vi "Main.vi"(11 "Module Admin":refnum<class "Delacor_lib_QMH_Cloneable Module Admin.lvclass">) -> ()   [LabVIEW 2021, in "MQTT Bridge.lvlib"]
doc: "This template is based off of the Queued Message Handler design pattern and the Queued Message Handler project template that ships with LabVIEW.\n\nThe main difference is that the queue is private to this module and communication between modules is performed via Broadcast and Request events.\n\nRequest events are wrapped in public API methods and are handled in the Event Handling Loop (EHL) of this VI. Any module can register for Broadcast events sent by this module. The EHL generates messages based on user interface actions.\n\nThe Message Handling Loop (MHL) processes messages generated by the EHL, or by other messages. The messages are string values, so new messages can be added easily to the Message Cases case structure in the MHL. Each message cluster can also provide an optional value for Message Data, which is a variant that can be converted to whatever message-specific data is required.\n_____\nBased on DQMH Dev Tools: Project Template 7.1.1.1528."
uses:
  MQTT Bridge.lvlib
  <vilib>/Delacor/Delacor QMH/Libraries/Cloneable Module Admin_class/Delacor_lib_QMH_Cloneable Module Admin.lvclass
  C:/Program Files (x86)/National Instruments/LabVIEW 2021/vi.lib/Delacor/Delacor QMH/Libraries/Module Admin_class/Delacor_lib_QMH_Module Admin.lvclass
  <vilib>/LabVIEW Open Source Project/MQTT Client/Client class/Client.lvclass/Client.ctl
  <vilib>/LabVIEW Open Source Project/MQTT Connection/MQTT_Base/Base Class/MQTT_Base.lvclass/MQTT_Base.ctl
  Module Data--cluster.ctl
  <vilib>/LabVIEW Open Source Project/MQTT Client/Client class/Client.lvclass
  C:/Program Files (x86)/National Instruments/LabVIEW 2021/vi.lib/LabVIEW Open Source Project/MQTT Connection/MQTT_Base/Base Class/MQTT_Base.lvclass
  <vilib>/Delacor/Delacor QMH/Libraries/Cloneable Module Admin_class/Delacor_lib_QMH_Cloneable Module Admin.lvclass/Delacor_lib_QMH_Cloneable Module Admin.ctl
  <vilib>/Delacor/Delacor QMH/Libraries/Message Queue_class/Delacor_lib_QMH_Message Queue.lvclass/Delacor_lib_QMH_Message Queue.ctl
  Stop Argument--cluster.ctl
  <vilib>/Delacor/Delacor QMH/Libraries/Module Admin_class/Delacor_lib_QMH_Module Admin.lvclass/Delacor_lib_QMH_Module Admin.ctl
  Connect Argument--cluster.ctl
  Subscribe Argument--cluster.ctl
  Subscribe (Reply Payload)--cluster.ctl
  Update Client Data Argument--cluster.ctl
  Disconnect Argument--cluster.ctl
  Check Connection Argument--cluster.ctl
  Check Connection (Reply Payload)--cluster.ctl
  Ack Variable Write Argument--cluster.ctl
  Ack Run Start Argument--cluster.ctl
  Get Recipe Argument--cluster.ctl
  Get Recipe (Reply Payload)--cluster.ctl
  Run Finished Argument--cluster.ctl
  Test Result Argument--cluster.ctl
  Test Result Payload.ctl
  <vilib>/Utility/miscctls.llb/LVPointTypeDef.ctl
  <vilib>/LabVIEW Open Source Project/MQTT Control Packets/Control Packets/CONNECT/ConnectFlags -- cluster.ctl
  <vilib>/Delacor/Delacor QMH/Libraries/Cloneable Module Admin_class/Delacor_lib_QMH_Get Module ID.vi
  <vilib>/Delacor/Delacor QMH/Libraries/Message Queue_class/Delacor_lib_QMH_Enqueue Message (Single).vi
  <vilib>/Delacor/Delacor QMH/Libraries/Module Admin_class/Delacor_lib_QMH_Get External Launch.vi
  6364ce0d-dd5e-4091-adf8-a46dd59fe2d6.vi
  d6dbc27b-4a7a-4a7a-b38d-2bf2a7d0c118.vi
  fed8d9bf-e88b-4754-9c8c-c458cda5f7ea.vi
  830f176a-2bba-44c1-832d-4bd8103bd494.vi
  <vilib>/JDP Science/JSONtext/Find Item.vi
  <vilib>/JDP Science/JSONtext/Next JSON Value.vi
  <vilib>/JDP Science/JSONtext/String Subset.vi
  <vilib>/JDP Science/JSONtext/Parsing/Advance past next JSON Value (inlined COPY).vi
  <vilib>/JDP Science/JSONtext/Parsing/Advance past whitespace.vi
  <vilib>/JDP Science/JSONtext/Parsing/Advance past String.vi
  <vilib>/JDP Science/JSONtext/Parsing/Advance past Number.vi
  <vilib>/JDP Science/JSONtext/Parsing/Advance past Line Ending.vi
  <vilib>/LabVIEW Open Source Project/Connection/Connection.TCP/Connection.TCP.lvclass
  C:/Program Files (x86)/National Instruments/LabVIEW 2021/vi.lib/LabVIEW Open Source Project/Connection/Connection/Connection.lvclass
  <vilib>/JDP Science/JSONtext/Parsing/Parse Full Path or Item Name.vi
  <vilib>/JDP Science/JSONtext/Parsing/Advance past Array.vi
  <vilib>/JDP Science/JSONtext/Parsing/Advance past Object.vi
  <vilib>/JDP Science/JSONtext/support/Error Cluster From Code.vi
  <vilib>/JDP Science/JSONtext/Offset/Find Item Locations by Path.vi
  <vilib>/JDP Science/JSONtext/JSON text to Variant.vi
  <vilib>/LabVIEW Open Source Project/MQTT Control Packets/Control Packets/PUBLISH/PUBLISH.lvclass
  <vilib>/JDP Science/JSONtext/LVClass Serializer/JSONtext LVClass Serializer.lvclass
  <vilib>/Delacor/Delacor QMH/Libraries/Message Queue_class/Delacor_lib_QMH_Message Queue.lvclass
  <vilib>/LabVIEW Open Source Project/MQTT Connection/MQTT_Base/Base Class/MQTT_Base.lvclass
  <vilib>/LabVIEW Open Source Project/MQTT Control Packets/Control Packets/CONNECT/CONNECT.lvclass
  C:/Program Files (x86)/National Instruments/LabVIEW 2021/vi.lib/LabVIEW Open Source Project/MQTT Client/Client class/Client.lvclass
  Sequence Engine/Modules/Sequence Engine/Sequence Engine.lvlib
panel:
  out "Topic":string
  out "payload":string
  out "error out":errorcluster
  out "Status":string
  in  "Simulate EHL Error":bool
  in  "Simulate MHL Error":bool
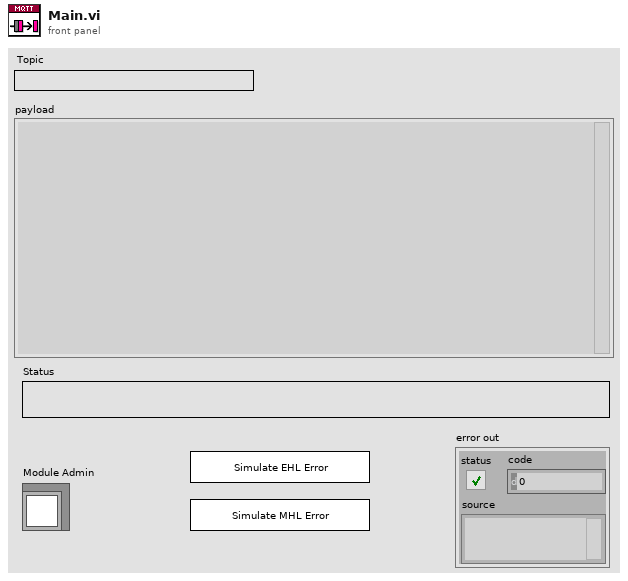
[diagram p1: front panel]
types:
  T1 = typedef "MQTT Client.lvlib/Client.lvclass/Public Events -- cluster.ctl" = cluster{"Connection Status":refnum<user-event>, "Connected":refnum<user-event>, "Application Message":refnum<user-event>}
  T2 = typedef "MQTT Base.lvlib/MQTT_Base.lvclass/Public Events -- cluster.ctl" = cluster{"Stop Event":refnum<user-event>, "Error Event":refnum<user-event>, "Inbound Message":refnum<user-event>}
  T3 = typedef "MQTT Bridge.lvlib/Request Events--cluster.ctl" = cluster{"Stop Module":refnum<user-event>, "Show Panel":refnum<user-event>, "Hide Panel":refnum<user-event>, "Show Diagram":refnum<user-event>, "Get Module Execution Status":refnum<user-event>, "Connect":refnum<user-event>, "Subscribe":refnum<user-event>, "Update Client Data":refnum<user-event>, "Disconnect":refnum<user-event>, "Check Connection":refnum<user-event>, "Ack Variable Write":refnum<user-event>, "Ack Run Start":refnum<user-event>, "Get Recipe":refnum<user-event>, "Run Finished":refnum<user-event>, "Test Result":refnum<user-event>}
  T4 = enum32{"invalid lock state", "Not Locked", "Locked (No Password)", "Password-protected"}
  T5 = typedef "MQTT Bridge.lvlib/Stop Argument--cluster.ctl" = cluster{"Module ID":i32, "Origin":string, "Exit via Stop Module Req?":bool, "Wait for Module to stop?":bool}
  T6 = typedef "MQTT Bridge.lvlib/Connect Argument--cluster.ctl" = cluster{"Module ID":i32, "Boolean":bool}
  T7 = typedef "MQTT Bridge.lvlib/Subscribe Argument--cluster.ctl" = cluster{"Module ID":i32, "Topic":string, "Wait Notifier":refnum<notifier>, "wait for reply":bool}
  T8 = typedef "MQTT Bridge.lvlib/Update Client Data Argument--cluster.ctl" = cluster{"Module ID":i32, "Client out":refnum<class "Client.lvclass">}
  T9 = typedef "MQTT Bridge.lvlib/Disconnect Argument--cluster.ctl" = cluster{"Module ID":i32, "Boolean":bool}
  T10 = typedef "MQTT Bridge.lvlib/Check Connection Argument--cluster.ctl" = cluster{"Module ID":i32, "Wait Notifier":refnum<notifier>, "wait for reply":bool}
  T11 = typedef "MQTT Bridge.lvlib/Ack Variable Write Argument--cluster.ctl" = cluster{"Module ID":i32, "JSON":string}
  T12 = typedef "MQTT Bridge.lvlib/Ack Run Start Argument--cluster.ctl" = cluster{"Module ID":i32, "JSON":string}
  T13 = typedef "MQTT Bridge.lvlib/Get Recipe Argument--cluster.ctl" = cluster{"Module ID":i32, "Get Recipe JSON":string, "Wait Notifier":refnum<notifier>, "wait for reply":bool}
  T14 = typedef "MQTT Bridge.lvlib/Run Finished Argument--cluster.ctl" = cluster{"Module ID":i32, "ts":dbl, "Run ID":string, "Result":string}
  T15 = typedef "MQTT Bridge.lvlib/Test Result Argument--cluster.ctl" = cluster{"Module ID":i32, "Test Result payload":T16}
  T16 = typedef "Test Result Payload.ctl" = cluster{"ts":dbl, "Run ID":string, "Test name":string, "Expected":string, "Measured":string, "Result":string, "Cycle Time_ms":u16}
  T17 = typedef "LVPointTypeDef.ctl" = cluster{"Horizontal":i16, "Vertical":i16}
  T18 = enum32{"Invalid", "Standard", "Closed", "Hidden", "Minimized", "Maximized"}
  T19 = typedef "MQTT_Control_Packets.lvlib/CONNECT.lvclass/ConnectFlags -- cluster.ctl" = cluster{"Reserved":bool, "Clean Session":bool, "Will Flag":bool, "Will QoS 1":bool, "Will QoS 2":bool, "Will Retain":bool, "Password Flag":bool, "User Name Flag":bool}
  T20 = typedef "MQTT Bridge.lvlib/Subscribe (Reply Payload)--cluster.ctl" = cluster{"Module ID":i32, "Subscribed":bool, "error":errorcluster}
  T21 = typedef "MQTT Bridge.lvlib/Check Connection (Reply Payload)--cluster.ctl" = cluster{"Module ID":i32, "Is Connected":bool, "error":errorcluster}
  T22 = typedef "MQTT Bridge.lvlib/Get Recipe (Reply Payload)--cluster.ctl" = cluster{"Module ID":i32, "Get Recipe reply JSON":string, "error":errorcluster}
  T23 = typedef "MQTT Bridge.lvlib/Module Data--cluster.ctl" = cluster{"MQTT_Base out":refnum<class "Client.lvclass">, "Status":string}
  T24 = typedef "MQTT_Control_Packets.lvlib/SUBSCRIBE.lvclass/Topic Subscription -- cluster.ctl" = cluster{"Topic Filter":string, "QoS":T25}
  T25 = typedef "MQTT_Control_Packets.lvlib/ControlPacket.lvclass/QualityOfService -- enum.ctl" = enum16{"0 (At Most Once)", "1 (At Least Once)", "2 (Exactly Once)"}
  T26 = typedef "MQTT_Control_Packets.lvlib/SUBACK.lvclass/Subscription Success Code.ctl" = cluster{"Subscription Failure":bool, "QoS":T25}
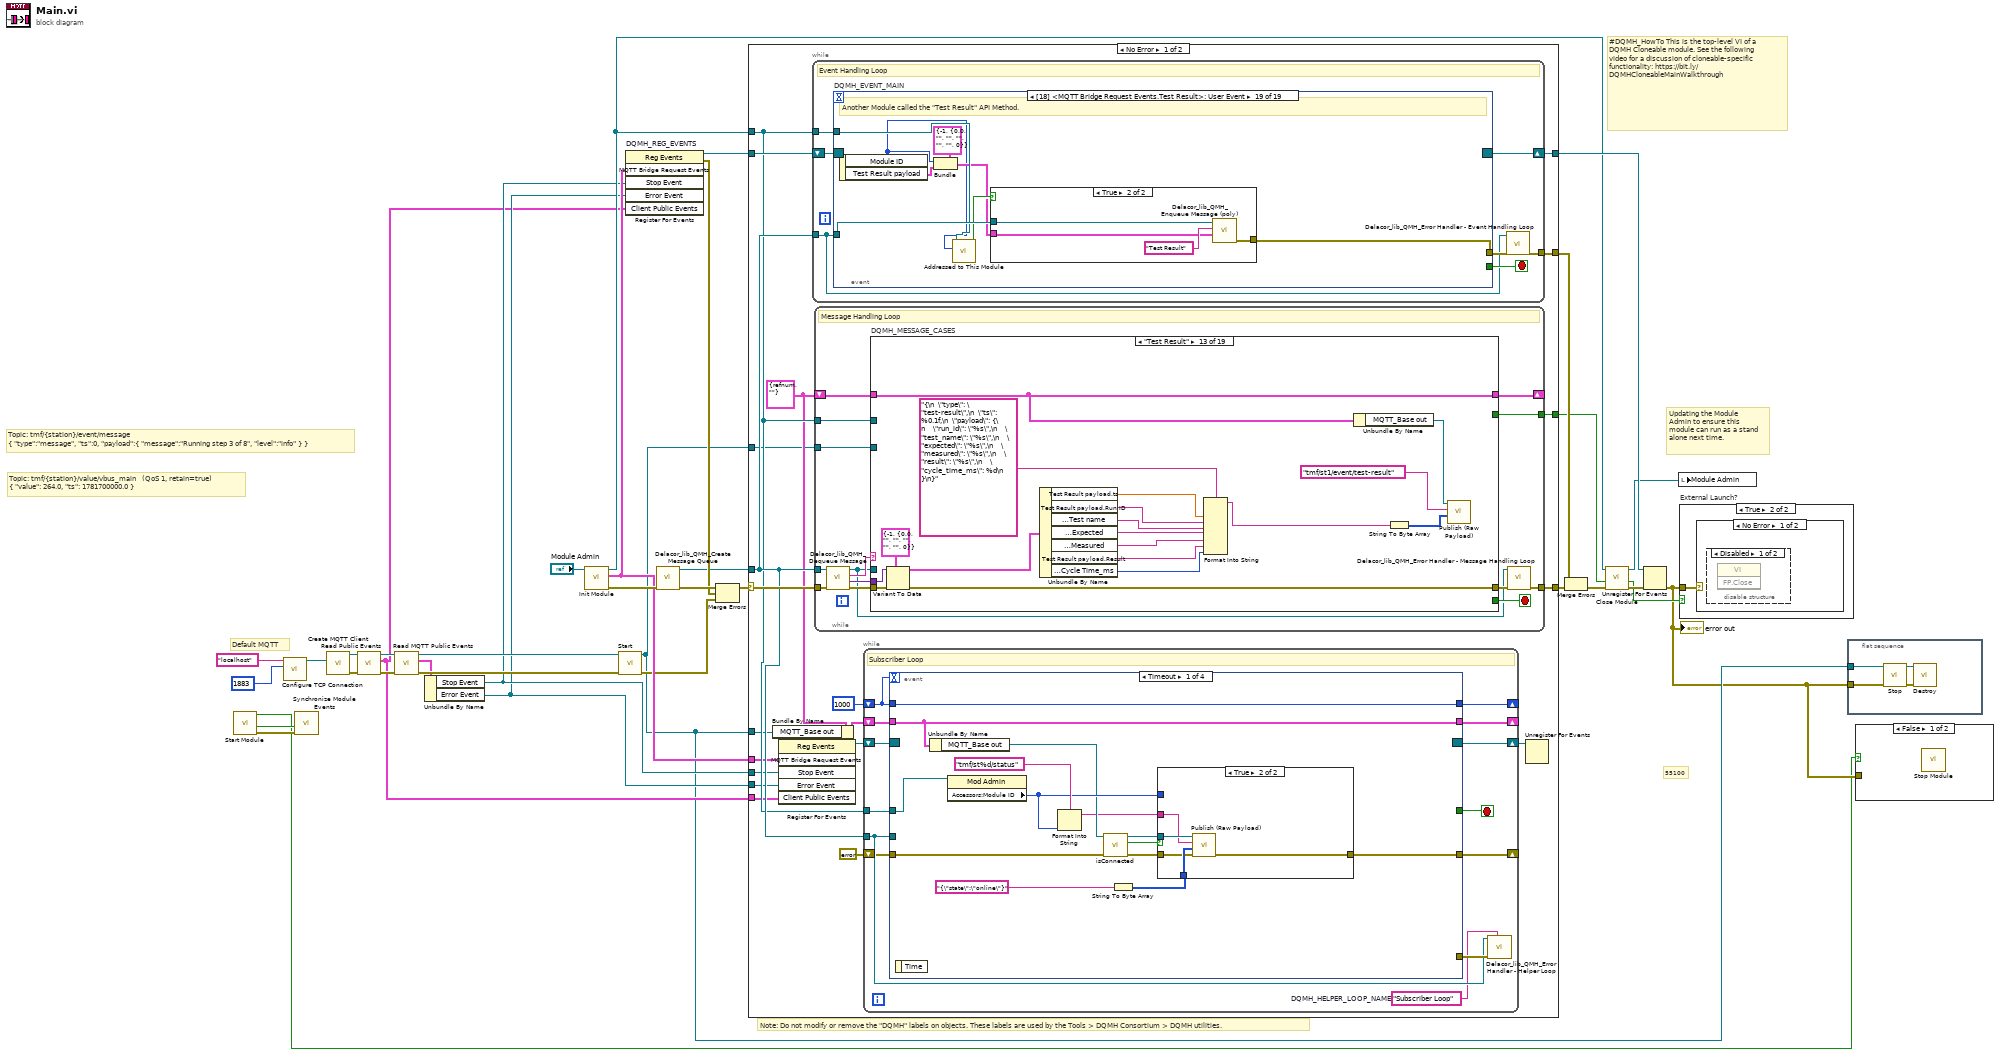
[diagram p0: block diagram]
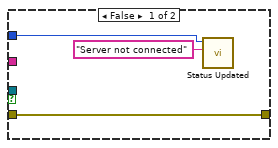
[diagram p3: hidden frame]
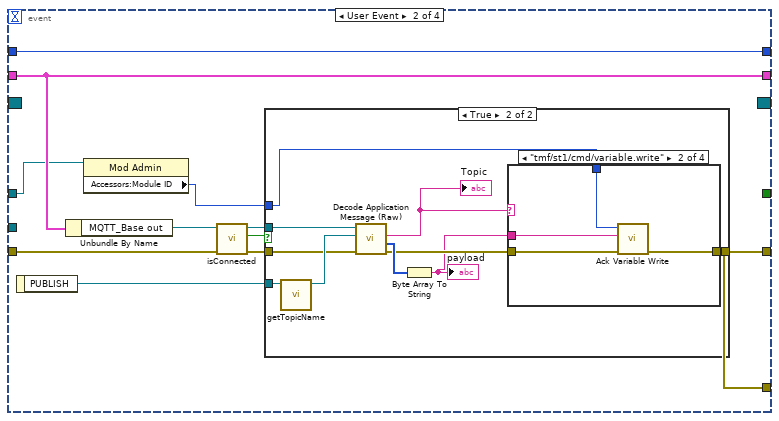
[diagram p4: hidden frame]
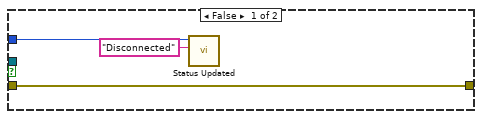
[diagram p5: hidden frame]
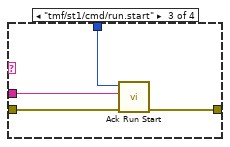
[diagram p7: hidden frame]
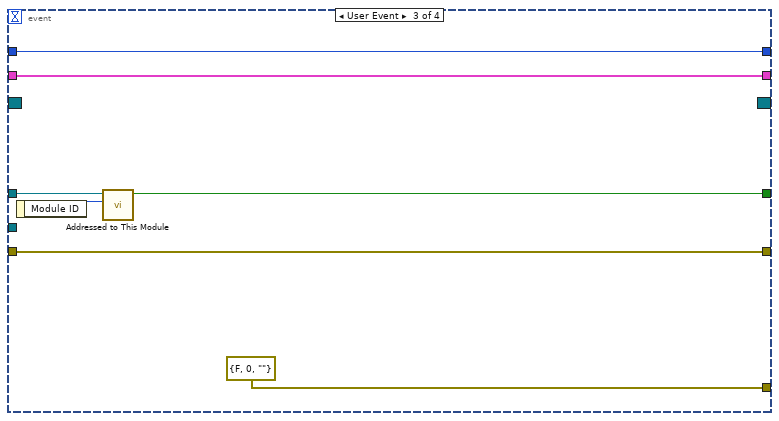
[diagram p9: hidden frame]
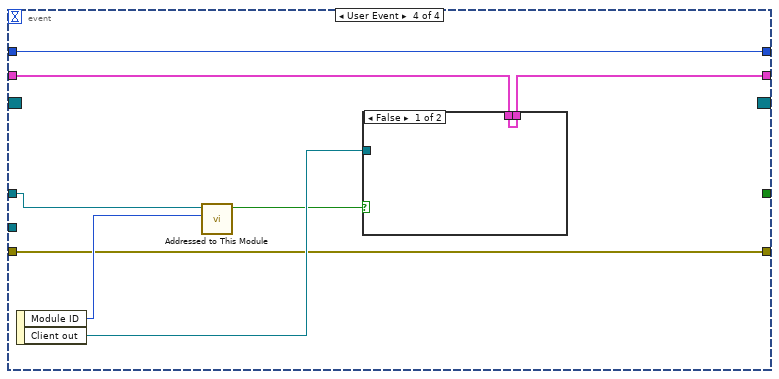
[diagram p10: hidden frame]
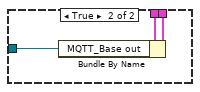
[diagram p11: hidden frame]
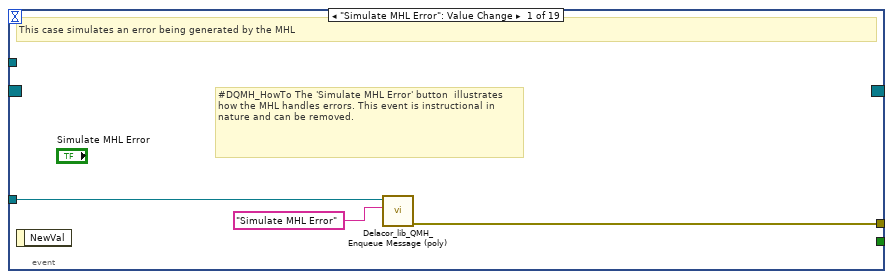
[diagram p12: hidden frame]
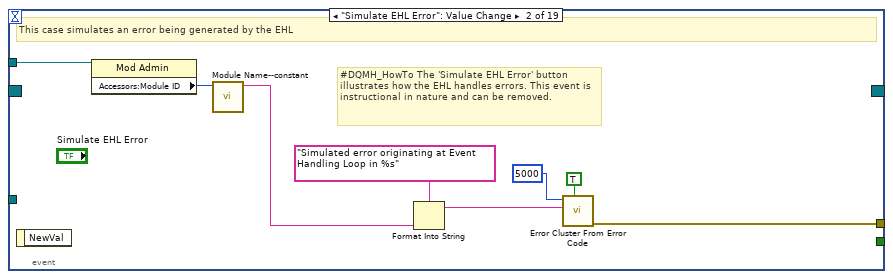
[diagram p13: hidden frame]
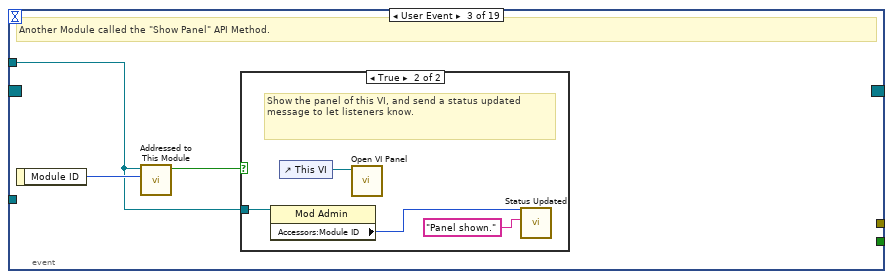
[diagram p14: hidden frame]
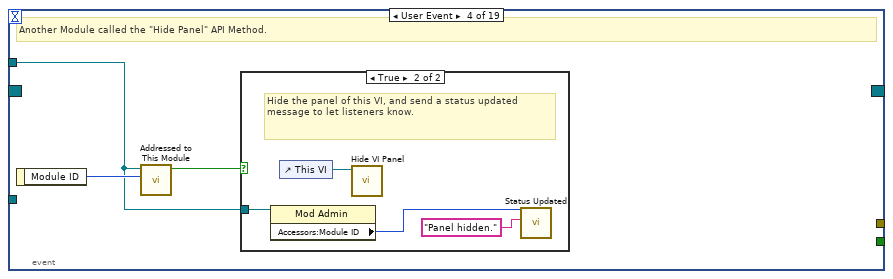
[diagram p16: hidden frame]
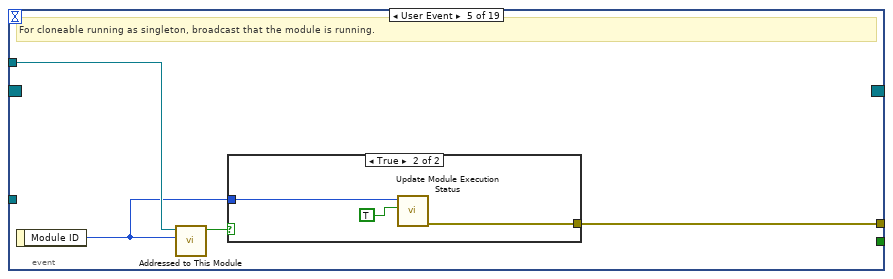
[diagram p18: hidden frame]
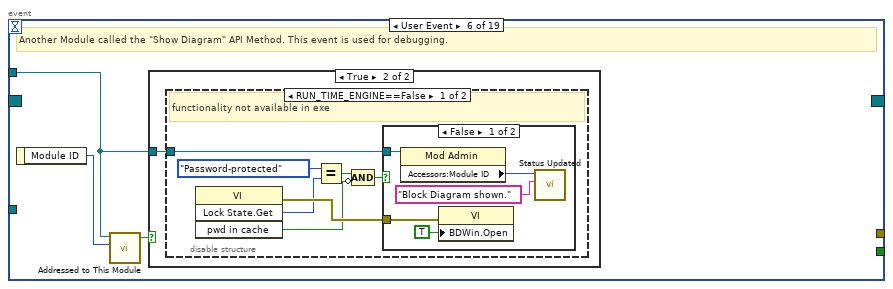
[diagram p20: hidden frame]
diagram:
  # "Topic: tmf/{station}/value/vbus_main   (QoS 1, retain=true)\n{ \"value\": 264.0, \"ts\": 1781700000.0 }"
  # "Topic: tmf/{station}/event/message\n{ \"type\":\"message\", \"ts\":0, \"payload\":{ \"message\":\"Running step 3 of 8\", \"level\":\"info\" } }"
  # "55100"
  # "Default MQTT"
  # "#DQMH_HowTo This is the top-level VI of a DQMH Cloneable module. See the following video for a discussion of cloneable-specific functionality: https://bit.ly/DQMHCloneableMainWalkthrough"
  # "Note: Do not modify or remove the \"DQMH\" labels on objects. These labels are used by the Tools > DQMH Consortium > DQMH utilities."
  # "Updating the Module Admin to ensure this module can run as a stand alone next time."
  n1 = call "Start Module.vi"() -> ("error out"=w4:errorcluster, "Wait for Event Sync?"=w3:bool, "Module Was Already Running?"=w1:bool)  [unwired: 7 in, 2 out]
  n2 = call <vilib>:"Configure TCP Connection.vi"("remote port (80)"=u16 1883, "address (localhost)"="localhost") -> ("Connection.TCP"=w19:refnum<class "Connection.TCP.lvclass">)  [unwired: 8 in, 1 out]
  n3 = call "Synchronize Module Events.vi"("error in"=w4, "Wait for Event Sync?"=w3) -> ()  [unwired: 9 in, 1 out]
  n4 = call <vilib>:"Create MQTT Client.vi"("Connection Configuration"=w19) -> ("error out"=w16:errorcluster, "Client out"=w18:refnum<class "Client.lvclass">)  [unwired: 9 in]
  n5 = call <vilib>:"Read Public Events.vi"("error in (no error)"=w16, "Client in"=w18) -> ("error out"=w15:errorcluster, "Client Public Events"=w6:T1, "Client out"=w17:refnum<class "Client.lvclass">)  [unwired: 7 in]
  n6 = call <vilib>:"Read MQTT Public Events.vi"("error in (no error)"=w15, "MQTT_Base in"=w17) -> ("error out"=w14:errorcluster, "MQTT Public Events"=w12:T2, "MQTT_Base out"=w13:refnum<class "Client.lvclass">)  [unwired: 7 in]
  n7 = Unbundle By Name(w12) -> ("Stop Event"=w8:refnum<user-event>, "Error Event"=w7:refnum<user-event>)
  n8 = call "Init Module.vi"("Cloneable Module Admin in"="Module Admin") -> ("error out"=w33:errorcluster, "MQTT Bridge Request Events"=w20:T3, "Cloneable Module Admin out"=w24:refnum<class "Delacor_lib_QMH_Cloneable Module Admin.lvclass">)  [unwired: 8 in]
  n9 = call <vilib>:"Start.vi"("error in (no error)"=w14, "MQTT_Base in"=w13) -> ("error out"=w9:errorcluster, "MQTT_Base out"=w5:refnum<class "Client.lvclass">)  [unwired: 7 in, 1 out]
  n10 = register-events "DQMH_REG_EVENTS"(w20, w8, w7, w6) -> (reference out=w27:refnum<event-registration>, error out=w29:errorcluster)  [unwired: 2 in]
  n11 = call <vilib>:"Delacor_lib_QMH_Create Message Queue.vi"("error in"=w33) -> ("error out"=w31:errorcluster, "Message Queue"=w26:refnum<class "Delacor_lib_QMH_Message Queue.lvclass">)  [unwired: 9 in]
  n12 = Merge Errors(w31, w29, w9) -> (w30:errorcluster)
  n13 = case shown="No Error" w30 {
    selector: w30 -> [w54 w672]
    tunnel: [w56 w671] -> w34
    tunnel: [w53 w670] -> w28
    tunnel: w27 -> [w52 w670]
    tunnel: w26 -> [w51 w663]
    tunnel: [w55 _] -> w35
    tunnel: w24 -> [w50 w666]
    tunnel: [w49 _] -> w22
    tunnel: w20 -> [w48 _]
    tunnel: w8 -> [w43 _]
    tunnel: w7 -> [w42 _]
    tunnel: w6 -> [w41 _]
    tunnel: w5 -> [w40 _]
    tunnel: w5 -> [w38 _]
    frame No Error {
      w44 = T23 {"MQTT_Base out"=refnum, "Status"=""} ("Data Cluster")
      n14 = Bundle By Name(cluster=w44, "MQTT_Base out"=w38) -> (w39:T23)
      n15 = register-events ("DQMH_HELPER_REGFOREVENTS")(w48, w43, w42, w41) -> (reference out=w46:refnum<event-registration>)  [unwired: 2 in, 1 out]
      n16 = while {
        tunnel: w51 -> [w145]
        shift-right: [w148] -> w53
        shift-left: w52 -> [w149]
        tunnel: [w150] -> w55
        tunnel: w50 -> [w146]
        stop <- w147 stop-if-true
        # "Event Handling Loop"
        n17 = event "DQMH_EVENT_MAIN" shown="[18] <MQTT Bridge Request Events.Test Result>: User Event" {
          selector: w149 -> [_ _ _ _ _ _ _ _ _ _ _ _ _ _ _ _ _ _ _]
          dyn-events: [_ _ _ _ _ _ _ _ _ _ _ _ _ _ _ _ _ _ _] -> w148
          timeout: _ -> [_ _ _ _ _ _ _ _ _ _ _ _ _ _ _ _ _ _ _]
          tunnel: [_ _ _ _ _ _ w203 _ _ _ _ _ _ _ _ _ _ _ _] -> w147
          tunnel: w145 -> [w153 _ _ _ _ _ w206 _ w226 w246 w260 w272 w284 w297 w309 w321 w335 w349 w361]
          tunnel: [w154 w162 _ _ w180 _ w207 w221 w229 w239 w251 w265 w277 w289 w302 w314 w326 w343 w354] -> w151
          tunnel: w146 -> [_ w161 w163 w170 w178 w184 w205 w223 w227 w244 w258 w270 w282 w295 w307 w319 w333 w347 w359]
          event "Simulate MHL Error": Value Change {
            # "#DQMH_HowTo The 'Simulate MHL Error' button  illustrates how the MHL handles errors. This event is instructional in nature and can be removed."
            # "This case simulates an error being generated by the MHL"
            n18 = event-data() -> ()  [unwired: 1 in, 1 out]
            n19 = call-poly <vilib>:"Delacor_lib_QMH_Enqueue Message (poly).vi"("Message"="Simulate MHL Error", "Message Queue in"=w153) -> ("error out"=w154:errorcluster)  [unwired: 8 in, 1 out]
          }
          event "Simulate EHL Error": Value Change {
            # "#DQMH_HowTo The 'Simulate EHL Error' button  illustrates how the EHL handles errors. This event is instructional in nature and can be removed."
            # "This case simulates an error being generated by the EHL"
            n20 = event-data() -> ()  [unwired: 1 in, 1 out]
            n21 = property on="Property Node" class="Mod Admin"(reference=w161) -> ("Accessors:Module ID"=w160:i32)  [unwired: 1 in, 2 out]
            n22 = call "Module Name--constant.vi"("Module ID"=w160) -> ("Module Name"=w155:string)  [unwired: 10 in]
            n23 = Format Into String(format string="Simulated error originating at Event Handling Loop in %s", w155) -> (resulting string=w158:string)  [unwired: 2 in, 1 out]
            n24 = call <vilib>:"Error Cluster From Error Code.vi"("show call chain? (False)"=TRUE, "error message (\"\")"=w158, "error code (0)"=5000) -> ("error out"=w162:errorcluster)  [unwired: 6 in]
          }
          event User Event {
            # "Another Module called the \"Show Panel\" API Method."
            n25 = event-data() -> ("Module ID"=w164:i32)  [unwired: 1 in]
            n26 = call "Addressed to This Module.vi"("Module ID from Argument"=w164, "Module Admin"=w163) -> ("Addressed to this instance?"=w165:bool)  [unwired: 8 in, 1 out]
            n27 = case shown="True" w165 {
              tunnel: w163 -> [_ w167]
              frame False {
              }
              frame True {
                # "Show the panel of this VI, and send a status updated message to let listeners know."
                n28 = property on="Property Node" class="Mod Admin"(reference=w167) -> ("Accessors:Module ID"=w166:i32)  [unwired: 1 in, 2 out]
                n29 = control-ref of="This VI"() -> (w169:refnum<vi>)
                n30 = call "Open VI Panel.vi"("VI"=w169) -> ()  [unwired: 10 in, 1 out]
                n31 = call "Status Updated.vi"("Status"="Panel shown." ("format string"), "Module ID"=w166) -> ()  [unwired: 9 in, 1 out]
              }
            }
          }
          event User Event {
            # "Another Module called the \"Hide Panel\" API Method."
            n32 = event-data() -> ("Module ID"=w171:i32)  [unwired: 1 in]
            n33 = call "Addressed to This Module.vi"("Module ID from Argument"=w171, "Module Admin"=w170) -> ("Addressed to this instance?"=w172:bool)  [unwired: 8 in, 1 out]
            n34 = case shown="True" w172 {
              tunnel: w170 -> [_ w174]
              frame False {
              }
              frame True {
                # "Hide the panel of this VI, and send a status updated message to let listeners know."
                n35 = property on="Property Node" class="Mod Admin"(reference=w174) -> ("Accessors:Module ID"=w173:i32)  [unwired: 1 in, 2 out]
                n36 = control-ref of="This VI"() -> (w176:refnum<vi>)
                n37 = call "Hide VI Panel.vi"("VI"=w176) -> ()  [unwired: 10 in, 1 out]
                n38 = call "Status Updated.vi"("Status"="Panel hidden." ("format string"), "Module ID"=w173) -> ()  [unwired: 9 in, 1 out]
              }
            }
          }
          event User Event {
            # "For cloneable running as singleton, broadcast that the module is running."
            n39 = event-data() -> ("Module ID"=w177:i32)  [unwired: 1 in]
            n40 = call "Addressed to This Module.vi"("Module ID from Argument"=w177, "Module Admin"=w178) -> ("Addressed to this instance?"=w179:bool)  [unwired: 8 in, 1 out]
            n41 = case shown="True" w179 {
              tunnel: [_ w183] -> w180
              tunnel: w177 -> [_ w182]
              frame False {
              }
              frame True {
                n42 = call "Update Module Execution Status.vi"("Running?"=TRUE, "Module ID"=w182) -> ("error out"=w183:errorcluster)  [unwired: 9 in]
              }
            }
          }
          event User Event {
            # "Another Module called the \"Show Diagram\" API Method. This event is used for debugging."
            n43 = event-data() -> ("Module ID"=w185:i32)  [unwired: 1 in]
            n44 = call "Addressed to This Module.vi"("Module ID from Argument"=w185, "Module Admin"=w184) -> ("Addressed to this instance?"=w186:bool)  [unwired: 8 in, 1 out]
            n45 = case shown="True" w186 {
              tunnel: w184 -> [_ w187]
              frame False {
              }
              frame True {
                n46 = disable-structure shown="RUN_TIME_ENGINE==False" {
                  disable-tunnel: w187 -> [w188 _]
                  frame condition #0 (active) {
                    # "functionality not available in exe"
                    n47 = invoke on="Invoke Node" class="VI" method="Lock State.Get"() -> (error out=w194:errorcluster, "Get Lock State"=w193:T4, "pwd in cache"=w190:bool)  [unwired: 4 in, 1 out]
                    n48 = Equal?(x=T4."Password-protected", y=w193) -> (x = y?=w191:bool)
                    n49 = Compound Arithmetic op=AND(w191, invert w190) -> (w189:bool)
                    n50 = case shown="False" w189 {
                      tunnel: w194 -> [w199 _]
                      tunnel: w188 -> [w196 _]
                      frame False {
                        n51 = property on="Property Node" class="Mod Admin"(reference=w196) -> ("Accessors:Module ID"=w195:i32)  [unwired: 1 in, 2 out]
                        n52 = property on="Property Node" class="VI"(error in=w199, "BDWin.Open"=TRUE ("Block Diagram Window:Open")) -> ()  [unwired: 1 in, 2 out]
                        n53 = call "Status Updated.vi"("Status"="Block Diagram shown." ("format string"), "Module ID"=w195) -> ()  [unwired: 9 in, 1 out]
                      }
                      frame True {
                        # "Password-protected VI, and the password is not in the cache. Do not show the diagram."
                      }
                    }
                  }
                  frame condition #1 {
                  }
                }
              }
            }
          }
          event User Event {
            # "Another Module called the \"Stop Module\" API Method  or the Message Handling Loop below."
            n54 = event-data() -> ("Module ID"=w201:i32, "Wait for Module to stop?"=w202:bool, "Origin"=w200:string)  [unwired: 1 in]
            n55 = call "Addressed to This Module.vi"("Module ID from Argument"=w201, "Module Admin"=w205) -> ("Addressed to this instance?"=w204:bool)  [unwired: 8 in, 1 out]
            n56 = case shown="True" w204 {
              tunnel: [_ w219] -> w207
              tunnel: w206 -> [_ w215]
              tunnel: [_ TRUE] -> w203
              tunnel: w202 -> [_ w210]
              tunnel: w201 -> [_ w212]
              tunnel: w200 -> [_ w208]
              frame False {
              }
              frame True {
                # "The event can get fired from the Exit message. The queue gets destroyed there. In this case, the Enqueue VI will return error 1. It is safe to ignore, because the module is already exiting."
                n57 = local write "Status"(w208) -> ()
                n58 = Bundle By Name(cluster=T5 {"Module ID"=-1, "Origin"="", "Exit via Stop Module Req?"=FALSE, "Wait for Module to stop?"=FALSE} ("Stop Argument"), "Module ID"=w212, "Exit via Stop Module Req?"=TRUE, "Wait for Module to stop?"=w210) -> (w209:T5)
                n59 = call-poly <vilib>:"Delacor_lib_QMH_Enqueue Message (poly).vi"("Priority Message? (F)"=TRUE, "Message Data"=w209, "Message"="Exit", "Message Queue in"=w215) -> ("error out"=w220:errorcluster)  [unwired: 6 in, 1 out]
                n60 = call <vilib>:"Clear Errors.vi"("error in (no error)"=w220, "specific error code to clear (0: all)"=1) -> ("error out"=w219:errorcluster)  [unwired: 4 in, 1 out]
              }
            }
          }
          event User Event {
            n61 = event-data() -> ()  [unwired: 1 in, 1 out]
            n62 = property class="Mod Admin"(reference=w223) -> ("Accessors:Module ID"=w222:i32)  [unwired: 1 in, 2 out]
            n63 = call "Stop Module.vi"("Module ID"=w222) -> ("error out"=w221:errorcluster)  [unwired: 10 in]
          }
          event Panel Close? {
            w228 = TRUE  # Discard the event, the MHL is responsible for closing and stopping this VI.
            # "Hide the panel or send the 'Exit' message if the user clicks the 'X' on the module main VI panel."
            n64 = event-data() -> ()  [unwired: 1 in, 1 out]
            n65 = property on="Property Node" class="Mod Admin"(reference=w227) -> (reference out=w224:refnum<class "Delacor_lib_QMH_Cloneable Module Admin.lvclass">, "Accessors:External Launch"=w225:bool)  [unwired: 1 in, 1 out]
            n66 = case shown="True" w225 {
              tunnel: w226 -> [_ w237]
              tunnel: [_ w238] -> w229
              tunnel: w224 -> [w232 _]
              frame True {
                # "If externally launched, clicking the 'X' hides the panel, but doesn't close it."
                n67 = property on="Property Node" class="Mod Admin"(reference=w232) -> ("Accessors:Module ID"=w231:i32)  [unwired: 1 in, 2 out]
                n68 = call "Status Updated.vi"("Status"="Panel hidden." ("format string"), "Module ID"=w231) -> ("error out"=w230:errorcluster)  [unwired: 9 in]
                n69 = control-ref of="This VI"() -> (w234:refnum<vi>)
                n70 = call "Hide VI Panel.vi"("error in"=w230, "VI"=w234) -> ()  [unwired: 9 in, 1 out]
              }
              frame False {
                # "If run as a stand-alone VI, clicking the panel 'X' stops the VI."
                n71 = call-poly <vilib>:"Delacor_lib_QMH_Enqueue Message (poly).vi"("Priority Message? (F)"=TRUE, "Message"="Exit", "Message Queue in"=w237) -> ("error out"=w238:errorcluster)  [unwired: 7 in, 1 out]
              }
            }
            n72 = event-data ("Event Filter Node")("Discard?"=w228) -> ()  [unwired: 1 in, 1 out]
          }
          event User Event {
            # "Another Module called the \"Connect\" API Method."
            n73 = event-data() -> ("Module ID"=w241:i32, "Boolean"=w240:bool)  [unwired: 1 in]
            n74 = Bundle(cluster=T6 {"Module ID"=-1, "Boolean"=FALSE} ("Connect Argument"), "Module ID"=w241, "Boolean"=w240) -> (w242:T6)
            n75 = call "Addressed to This Module.vi"("Module ID from Argument"=w241, "Module Admin"=w244) -> ("Addressed to this instance?"=w245:bool)  [unwired: 8 in, 1 out]
            n76 = case shown="True" w245 {
              tunnel: w246 -> [_ w250]
              tunnel: w242 -> [_ w248]
              tunnel: [_ w247] -> w239
              frame False {
              }
              frame True {
                n77 = call-poly <vilib>:"Delacor_lib_QMH_Enqueue Message (poly).vi"("Message Data"=w248, "Message"="Connect", "Message Queue in"=w250) -> ("error out"=w247:errorcluster)  [unwired: 7 in, 1 out]
              }
            }
          }
          event User Event {
            # "Another Module called the \"Subscribe\" API Method."
            n78 = event-data() -> ("Module ID"=w255:i32, "Topic"=w254:string, "Wait Notifier"=w253:refnum<notifier>, "wait for reply"=w252:bool)  [unwired: 1 in]
            n79 = Bundle(cluster=T7 {"Module ID"=-1, "Topic"="", "Wait Notifier"=refnum, "wait for reply"=FALSE} ("Subscribe Argument"), "Module ID"=w255, "Topic"=w254, "Wait Notifier"=w253, "wait for reply"=w252) -> (w256:T7)
            n80 = call "Addressed to This Module.vi"("Module ID from Argument"=w255, "Module Admin"=w258) -> ("Addressed to this instance?"=w259:bool)  [unwired: 8 in, 1 out]
            n81 = case shown="True" w259 {
              tunnel: w260 -> [_ w264]
              tunnel: w256 -> [_ w262]
              tunnel: [_ w261] -> w251
              frame False {
              }
              frame True {
                n82 = call-poly <vilib>:"Delacor_lib_QMH_Enqueue Message (poly).vi"("Message Data"=w262, "Message"="Subscribe", "Message Queue in"=w264) -> ("error out"=w261:errorcluster)  [unwired: 7 in, 1 out]
              }
            }
          }
          event User Event {
            # "Another Module called the \"Update Client Data\" API Method."
            n83 = event-data() -> ("Module ID"=w267:i32, "Client out"=w266:refnum<class "Client.lvclass">)  [unwired: 1 in]
            n84 = Bundle(cluster=T8 {"Module ID"=-1, "Client out"=refnum} ("Update Client Data Argument"), "Module ID"=w267, "Client out"=w266) -> (w268:T8)
            n85 = call "Addressed to This Module.vi"("Module ID from Argument"=w267, "Module Admin"=w270) -> ("Addressed to this instance?"=w271:bool)  [unwired: 8 in, 1 out]
            n86 = case shown="True" w271 {
              tunnel: w272 -> [_ w276]
              tunnel: w268 -> [_ w274]
              tunnel: [_ w273] -> w265
              frame False {
              }
              frame True {
                n87 = call-poly <vilib>:"Delacor_lib_QMH_Enqueue Message (poly).vi"("Message Data"=w274, "Message"="Update Client Data", "Message Queue in"=w276) -> ("error out"=w273:errorcluster)  [unwired: 7 in, 1 out]
              }
            }
          }
          event User Event {
            # "Another Module called the \"Disconnect\" API Method."
            n88 = event-data() -> ("Module ID"=w279:i32, "Boolean"=w278:bool)  [unwired: 1 in]
            n89 = Bundle(cluster=T9 {"Module ID"=-1, "Boolean"=FALSE} ("Disconnect Argument"), "Module ID"=w279, "Boolean"=w278) -> (w280:T9)
            n90 = call "Addressed to This Module.vi"("Module ID from Argument"=w279, "Module Admin"=w282) -> ("Addressed to this instance?"=w283:bool)  [unwired: 8 in, 1 out]
            n91 = case shown="True" w283 {
              tunnel: w284 -> [_ w288]
              tunnel: w280 -> [_ w286]
              tunnel: [_ w285] -> w277
              frame False {
              }
              frame True {
                n92 = call-poly <vilib>:"Delacor_lib_QMH_Enqueue Message (poly).vi"("Message Data"=w286, "Message"="Disconnect", "Message Queue in"=w288) -> ("error out"=w285:errorcluster)  [unwired: 7 in, 1 out]
              }
            }
          }
          event User Event {
            # "Another Module called the \"Check Connection\" API Method."
            n93 = event-data() -> ("Module ID"=w292:i32, "Wait Notifier"=w291:refnum<notifier>, "wait for reply"=w290:bool)  [unwired: 1 in]
            n94 = Bundle(cluster=T10 {"Module ID"=-1, "Wait Notifier"=refnum, "wait for reply"=FALSE} ("Check Connection Argument"), "Module ID"=w292, "Wait Notifier"=w291, "wait for reply"=w290) -> (w293:T10)
            n95 = call "Addressed to This Module.vi"("Module ID from Argument"=w292, "Module Admin"=w295) -> ("Addressed to this instance?"=w296:bool)  [unwired: 8 in, 1 out]
            n96 = case shown="True" w296 {
              tunnel: w297 -> [_ w301]
              tunnel: w293 -> [_ w299]
              tunnel: [_ w298] -> w289
              frame False {
              }
              frame True {
                n97 = call-poly <vilib>:"Delacor_lib_QMH_Enqueue Message (poly).vi"("Message Data"=w299, "Message"="Check Connection", "Message Queue in"=w301) -> ("error out"=w298:errorcluster)  [unwired: 7 in, 1 out]
              }
            }
          }
          event User Event {
            # "Another Module called the \"Ack Variable Write\" API Method."
            n98 = event-data() -> ("Module ID"=w304:i32, "JSON"=w303:string)  [unwired: 1 in]
            n99 = Bundle(cluster=T11 {"Module ID"=-1, "JSON"=""} ("Ack Variable Write Argument"), "Module ID"=w304, "JSON"=w303) -> (w305:T11)
            n100 = call "Addressed to This Module.vi"("Module ID from Argument"=w304, "Module Admin"=w307) -> ("Addressed to this instance?"=w308:bool)  [unwired: 8 in, 1 out]
            n101 = case shown="True" w308 {
              tunnel: w309 -> [_ w313]
              tunnel: w305 -> [_ w311]
              tunnel: [_ w310] -> w302
              frame False {
              }
              frame True {
                n102 = call-poly <vilib>:"Delacor_lib_QMH_Enqueue Message (poly).vi"("Message Data"=w311, "Message"="Ack Variable Write", "Message Queue in"=w313) -> ("error out"=w310:errorcluster)  [unwired: 7 in, 1 out]
              }
            }
          }
          event User Event {
            # "Another Module called the \"Ack Run Start\" API Method."
            n103 = event-data() -> ("Module ID"=w316:i32, "JSON"=w315:string)  [unwired: 1 in]
            n104 = Bundle(cluster=T12 {"Module ID"=-1, "JSON"=""} ("Ack Run Start Argument"), "Module ID"=w316, "JSON"=w315) -> (w317:T12)
            n105 = call "Addressed to This Module.vi"("Module ID from Argument"=w316, "Module Admin"=w319) -> ("Addressed to this instance?"=w320:bool)  [unwired: 8 in, 1 out]
            n106 = case shown="True" w320 {
              tunnel: w321 -> [_ w325]
              tunnel: w317 -> [_ w323]
              tunnel: [_ w322] -> w314
              frame False {
              }
              frame True {
                n107 = call-poly <vilib>:"Delacor_lib_QMH_Enqueue Message (poly).vi"("Message Data"=w323, "Message"="Ack Run Start", "Message Queue in"=w325) -> ("error out"=w322:errorcluster)  [unwired: 7 in, 1 out]
              }
            }
          }
          event User Event {
            # "Another Module called the \"Get Recipe\" API Method."
            n108 = event-data() -> ("Module ID"=w330:i32, "Get Recipe JSON"=w329:string, "Wait Notifier"=w328:refnum<notifier>, "wait for reply"=w327:bool)  [unwired: 1 in]
            n109 = Bundle(cluster=T13 {"Module ID"=-1, "Get Recipe JSON"="", "Wait Notifier"=refnum, "wait for reply"=FALSE} ("Get Recipe Argument"), "Module ID"=w330, "Get Recipe JSON"=w329, "Wait Notifier"=w328, "wait for reply"=w327) -> (w331:T13)
            n110 = call "Addressed to This Module.vi"("Module ID from Argument"=w330, "Module Admin"=w333) -> ("Addressed to this instance?"=w334:bool)  [unwired: 8 in, 1 out]
            n111 = case shown="True" w334 {
              tunnel: w335 -> [_ w339]
              tunnel: w331 -> [_ w337]
              tunnel: [_ w336] -> w326
              frame False {
              }
              frame True {
                n112 = call-poly <vilib>:"Delacor_lib_QMH_Enqueue Message (poly).vi"("Message Data"=w337, "Message"="Get Recipe", "Message Queue in"=w339) -> ("error out"=w336:errorcluster)  [unwired: 7 in, 1 out]
              }
            }
          }
          event User Event {
            # "Another Module called the \"Run Finished\" API Method."
            n113 = event-data() -> ("Module ID"=w344:i32, "ts"=w342:dbl, "Run ID"=w341:string, "Result"=w340:string)  [unwired: 1 in]
            n114 = Bundle(cluster=T14 {"Module ID"=-1, "ts"=0.0, "Run ID"="", "Result"=""} ("Run Finished Argument"), "Module ID"=w344, "ts"=w342, "Run ID"=w341, "Result"=w340) -> (w345:T14)
            n115 = call "Addressed to This Module.vi"("Module ID from Argument"=w344, "Module Admin"=w347) -> ("Addressed to this instance?"=w348:bool)  [unwired: 8 in, 1 out]
            n116 = case shown="True" w348 {
              tunnel: w349 -> [_ w353]
              tunnel: w345 -> [_ w351]
              tunnel: [_ w350] -> w343
              frame False {
              }
              frame True {
                n117 = call-poly <vilib>:"Delacor_lib_QMH_Enqueue Message (poly).vi"("Message Data"=w351, "Message"="Run Finished", "Message Queue in"=w353) -> ("error out"=w350:errorcluster)  [unwired: 7 in, 1 out]
              }
            }
          }
          event User Event {
            # "Another Module called the \"Test Result\" API Method."
            n118 = event-data() -> ("Module ID"=w356:i32, "Test Result payload"=w355:T16)  [unwired: 1 in]
            n119 = Bundle(cluster=T15 {"Module ID"=-1, "Test Result payload"={"ts"=0.0, "Run ID"="", "Test name"="", "Expected"="", "Measured"="", "Result"="", "Cycle Time_ms"=0}} ("Test Result Argument"), "Module ID"=w356, "Test Result payload"=w355) -> (w357:T15)
            n120 = call "Addressed to This Module.vi"("Module ID from Argument"=w356, "Module Admin"=w359) -> ("Addressed to this instance?"=w360:bool)  [unwired: 8 in, 1 out]
            n121 = case shown="True" w360 {
              tunnel: w361 -> [_ w365]
              tunnel: w357 -> [_ w363]
              tunnel: [_ w362] -> w354
              frame False {
              }
              frame True {
                n122 = call-poly <vilib>:"Delacor_lib_QMH_Enqueue Message (poly).vi"("Message Data"=w363, "Message"="Test Result", "Message Queue in"=w365) -> ("error out"=w362:errorcluster)  [unwired: 7 in, 1 out]
              }
            }
          }
        }
        n123 = call-dynamic "Delacor_lib_QMH_Error Handler - Event Handling Loop.vi"("error in"=w151, "Message Queue in"=w145) -> ("dup error in"=w150:errorcluster)  [unwired: 8 in, 1 out]
      }
      n124 = while {
        tunnel: w51 -> [w367]
        shift-right: [w374] -> _
        shift-left: w44 -> [w375]
        tunnel: w54 -> [w378]
        tunnel: [w376] -> w56
        tunnel: w50 -> [w369]
        tunnel: [w368] -> w49
        tunnel: w40 -> [w366]
        stop <- w373 stop-if-true
        # "Message Handling Loop"
        n125 = call-dynamic "Delacor_lib_QMH_Dequeue Message.vi"("error in"=w378, "Message Queue in"=w367) -> ("error out"=w377:errorcluster, "Message Data"=w371:variant, "Message"=w372:string, "Message Queue out"=w370:refnum<class "Delacor_lib_QMH_Message Queue.lvclass">)  [unwired: 6 in]
        n126 = case "DQMH_MESSAGE_CASES" shown="\"Test Result\"" w372 {
          selector: w372 -> [_ _ _ _ _ _ _ _ _ _ _ _ _ _ _ _ _ _ w652]
          tunnel: w370 -> [_ _ w406 _ _ _ _ _ _ _ _ _ _ _ _ w607 _ w644 _]
          tunnel: w377 -> [w399 w403 w423 w437 w466 w476 w490 w509 w528 w546 w562 w581 w599 w602 w604 w616 w633 w650 w661]
          tunnel: [w397 w403 w405 w437 w458 w474 w481 w501 w527 w545 w554 w580 w598 w601 w604 w612 w632 w645 w662] -> w379
          tunnel: w375 -> [w390 w402 w419 w435 w456 w475 w483 w492 w519 w532 w550 w573 w589 w600 w603 w611 w630 w643 w659]
          tunnel: [w389 w402 w419 w435 w456 w470 w483 w492 w519 w532 w550 w573 w589 w600 w603 w611 w630 w643 w659] -> w374
          tunnel: [_ _ _ _ _ _ _ _ _ _ _ _ _ _ _ _ _ w642 _] -> w373
          tunnel: w371 -> [_ _ w422 _ w465 w473 w489 w508 w526 w544 w560 w579 w597 _ _ w610 _ w640 _]
          tunnel: w369 -> [w385 _ w409 w436 w457 _ _ w500 _ _ w552 _ _ _ _ w609 w628 w635 w658]
          tunnel: [_ _ _ _ _ _ _ _ _ _ _ _ _ _ _ _ _ w638 _] -> w368
          tunnel: w366 -> [w380 _ _ _ _ _ _ _ _ _ _ _ _ _ _ _ _ _ _]
          frame "Initialize" {
            w382 = "Initial Message" ("Initial Message")
            # "Initialize - Any operation that needs to be done before the module can receive messages. Synchronize Caller Events.vi will inform Start Module.vi that the module has launched and is ready to receive messages. Module Did Init.vi will broadcast that the module initialized."
            n127 = call "Synchronize Caller Events.vi"("error in"=w399, "Module Admin"=w385) -> ("error out"=w398:errorcluster, "Module Admin out"=w384:refnum<class "Delacor_lib_QMH_Cloneable Module Admin.lvclass">)  [unwired: 8 in]
            n128 = property on="Property Node" class="Mod Admin"(reference=w384) -> ("Accessors:Module ID"=w381:i32, "Accessors:External Launch"=w386:bool)  [unwired: 1 in, 2 out]
            n129 = call "Module Name--constant.vi"("Module ID"=w381) -> ("Module Name"=w394:string)  [unwired: 10 in]
            n130 = property on="Property Node" class="VI"("Front Panel.Title"=w394) -> (reference out=w396:refnum<vi>, error out=w401:errorcluster)  [unwired: 2 in]
            n131 = Select(t=T18."Hidden" ("State"), s=w386, f=T18."Standard" ("State")) -> (s? t:f=w391:T18)
            n132 = Bundle By Name(cluster=w390, "MQTT_Base out"=w380, "Status"=w382) -> (w389:T23)
            n133 = invoke on="Invoke Node" class="VI" method="FP.Open"(reference=w396, error in=w401, "State"=w391) -> (reference out=w395:refnum<vi>, error out=w400:errorcluster)  [unwired: 2 in, 3 out]
            n134 = invoke on="Invoke Node" class="VI" method="FP.Center"(reference=w395, error in=w400) -> ()  [unwired: 1 in, 3 out]
            n135 = property on="Pane" class="Pane"("Origin"=T17 {"Horizontal"=0, "Vertical"=0}) -> ()  [unwired: 2 in, 2 out]
            n136 = call "Module Name--constant.vi"("Module ID"=w381) -> ("Module Name"=w387:string)  [unwired: 10 in]
            n137 = call "Module Did Init.vi"("error in"=w398, "Initialized?"=TRUE, "Origin"=w387, "Module ID"=w381) -> ("error out"=w397:errorcluster)  [unwired: 7 in]
            "Status" <- w382
          }
          frame "---Module Specific---" {
            # "Separator -- The following cases handle messages specific to this Module."
          }
          frame "Connect" {
            n138 = Variant To Data(error in=w423, type=T6 {"Module ID"=-1, "Boolean"=FALSE} ("Connect Argument"), Variant=w422) -> (data=w420:T6, error out=w416:errorcluster)
            n139 = Unbundle By Name(w420) -> ()  [unwired: 2 out]
            n140 = Unbundle By Name(w419) -> ("MQTT_Base out"=w418:refnum<class "Client.lvclass">)
            n141 = property class="Mod Admin"(reference=w409) -> ("Accessors:Module ID"=w408:i32)  [unwired: 1 in, 2 out]
            n142 = call <vilib>:"Connect to Server.vi"("Connect Flags"=T19 {"Reserved"=FALSE, "Clean Session"=TRUE, "Will Flag"=FALSE, "Will QoS 1"=FALSE, "Will QoS 2"=FALSE, "Will Retain"=FALSE, "Password Flag"=FALSE, "User Name Flag"=FALSE}, "error in (no error)"=w416, "Client in"=w418) -> ("error out"=w415:errorcluster, "Client out"=w414:refnum<class "Client.lvclass">)  [unwired: 5 in, 2 out]
            n143 = call <vilib>:"isConnected.vi"("error in (no error)"=w415, "Client in"=w414) -> ("connected"=w404:bool, "Client out"=w413:refnum<class "Client.lvclass">)  [unwired: 7 in, 1 out]
            n144 = call "Update Client Data.vi"("Client out"=w413, "Module ID"=w408) -> ("error out"=w407:errorcluster)  [unwired: 9 in]
            n145 = case shown="False" w404 {
              tunnel: w407 -> [w424 w428]
              tunnel: w406 -> [_ w427]
              tunnel: [w424 w425] -> w405
              frame False {
              }
              frame True {
                n146 = call-poly <vilib>:"Delacor_lib_QMH_Enqueue Message (poly).vi"("error in"=w428, "Message"="Subscribe bulk topics", "Message Queue in"=w427) -> ("error out"=w425:errorcluster)  [unwired: 7 in, 1 out]
              }
            }
            n147 = Select(t="Connected" ("Status"), s=w404, f="Connection failed") -> (s? t:f=w412:string)
            n148 = call "Status Updated.vi"("Status"=w412, "Module ID"=w408) -> ()  [unwired: 9 in, 1 out]
          }
          frame "Subscribe bulk topics" {
            n149 = property class="Mod Admin"(reference=w436) -> ("Accessors:Module ID"=w431:i32)  [unwired: 1 in, 2 out]
            n150 = Unbundle By Name(w435) -> ("MQTT_Base out"=w434:refnum<class "Client.lvclass">)
            n151 = call "Get Subscription Topics.vi"() -> ("Topic Subscriptions"=w429:T24[])  [unwired: 11 in]
            n152 = call <vilib>:"Subscribe (Array).vi"("Topic Subscriptions"=w429, "Client in"=w434) -> ("error out"=w433:errorcluster, "Subscription Success"=w430:T26[], "Client out"=w432:refnum<class "Client.lvclass">)  [unwired: 7 in]
            n153 = for {
              tunnel: w431 -> [w447]
              tunnel: w430 -> [w446] mode=indexing
              tunnel: w429 -> [w445] mode=indexing
              n154 = Unbundle By Name(w446) -> ("Subscription Failure"=w444:bool)
              n155 = Unbundle By Name(w445) -> ("Topic Filter"=w438:string)
              n156 = Format Into String(format string="Subs: %s", w438) -> (resulting string=w440:string)  [unwired: 2 in, 1 out]
              n157 = Format Into String(format string="Not Subs: %s", w438) -> (resulting string=w442:string)  [unwired: 2 in, 1 out]
              n158 = Select(t=w442, s=w444, f=w440) -> (s? t:f=w439:string)
              n159 = call "Status Updated.vi"("Status"=w439, "Module ID"=w447) -> ()  [unwired: 9 in, 1 out]
            }
            n160 = call "Update Client Data.vi"("error in"=w433, "Client out"=w432, "Module ID"=w431) -> ()  [unwired: 8 in, 1 out]
          }
          frame "Subscribe" {
            n161 = property class="Mod Admin"(reference=w457) -> ("Accessors:Module ID"=w449:i32)  [unwired: 1 in, 2 out]
            n162 = Variant To Data(error in=w466, type=T7 {"Module ID"=-1, "Topic"="", "Wait Notifier"=refnum, "wait for reply"=FALSE} ("Subscribe Argument"), Variant=w465) -> (data=w463:T7, error out=w452:errorcluster)
            n163 = Unbundle By Name(w463) -> ("Topic"=w454:string, "Wait Notifier"=w462:refnum<notifier>, "wait for reply"=w461:bool)  [unwired: 1 out]
            n164 = Unbundle By Name(w456) -> ("MQTT_Base out"=w455:refnum<class "Client.lvclass">)
            n165 = call <vilib>:"Subscribe (Scalar).vi"("error in (no error)"=w452, "Topic Filter"=w454, "Client in"=w455) -> ("error out"=w451:errorcluster, "Ack"=w453:bool, "Client out"=w448:refnum<class "Client.lvclass">)  [unwired: 6 in]
            n166 = call "Update Client Data.vi"("error in"=w451, "Client out"=w448, "Module ID"=w449) -> ("error out"=w450:errorcluster)  [unwired: 8 in]
            n167 = Bundle By Name(cluster=T20 {"Module ID"=-1, "Subscribed"=FALSE, "error"={"status"=FALSE, "code"=0, "source"=""}} ("Subscribe (Reply Payload)"), "Module ID"=w449, "Subscribed"=w453, "error"=w450) -> (w460:T20)
            n168 = Merge Errors(w452, w450) -> (w458:errorcluster)
            n169 = case "DQMH_FIRE_NOTIFIER" shown="True" w461 {
              tunnel: w462 -> [_ w468]
              tunnel: w460 -> [_ w467]
              frame False {
              }
              frame True {
                n170 = Send Notification(notification=w467, notifier=w468) -> ()  [unwired: 1 in, 2 out]
              }
            }
          }
          frame "Update Client Data" {
            n171 = Variant To Data(error in=w476, type=T8 {"Module ID"=-1, "Client out"=refnum} ("Update Client Data Argument"), Variant=w473) -> (data=w471:T8, error out=w474:errorcluster)
            n172 = Unbundle By Name(w471) -> ("Client out"=w469:refnum<class "Client.lvclass">)  [unwired: 1 out]
            n173 = Bundle By Name(cluster=w475, "MQTT_Base out"=w469) -> (w470:T23)
          }
          frame "Disconnect" {
            n174 = Variant To Data(error in=w490, type=T9 {"Module ID"=-1, "Boolean"=FALSE} ("Disconnect Argument"), Variant=w489) -> (data=w487:T9, error out=w481:errorcluster)
            n175 = Unbundle By Name(w487) -> ("Module ID"=w478:i32)  [unwired: 1 out]
            n176 = Unbundle By Name(w483) -> ("MQTT_Base out"=w482:refnum<class "Client.lvclass">)
            n177 = call <vilib>:"Disconnect from Server.vi"("error in (no error)"=w481, "Client in"=w482) -> ("error out"=w480:errorcluster, "Client out"=w477:refnum<class "Client.lvclass">)  [unwired: 7 in, 1 out]
            n178 = call "Update Client Data.vi"("error in"=w480, "Client out"=w477, "Module ID"=w478) -> ("error out"=w479:errorcluster)  [unwired: 8 in]
            n179 = Select(t="Error while disconnection" ("f"), s=w479, f="Disconnected" ("Status")) -> (s? t:f=w486:string)
            n180 = call "Status Updated.vi"("Status"=w486, "Module ID"=w478) -> ()  [unwired: 9 in, 1 out]
          }
          frame "Check Connection" {
            n181 = property class="Mod Admin"(reference=w500) -> ("Accessors:Module ID"=w495:i32)  [unwired: 1 in, 2 out]
            n182 = Variant To Data(error in=w509, type=T10 {"Module ID"=-1, "Wait Notifier"=refnum, "wait for reply"=FALSE} ("Check Connection Argument"), Variant=w508) -> (data=w506:T10, error out=w499:errorcluster)
            n183 = Unbundle By Name(w506) -> ("Wait Notifier"=w505:refnum<notifier>, "wait for reply"=w504:bool)  [unwired: 1 out]
            n184 = Unbundle By Name(w492) -> ("MQTT_Base out"=w491:refnum<class "Client.lvclass">)
            n185 = call <vilib>:"isConnected.vi"("error in (no error)"=w499, "Client in"=w491) -> ("error out"=w493:errorcluster, "connected"=w494:bool)  [unwired: 7 in, 1 out]
            n186 = Select(t="Connected" ("Status"), s=w494, f="Not Connected") -> (s? t:f=w498:string)
            n187 = call "Status Updated.vi"("Status"=w498, "Module ID"=w495) -> ()  [unwired: 9 in, 1 out]
            n188 = Bundle By Name(cluster=T21 {"Module ID"=-1, "Is Connected"=FALSE, "error"={"status"=FALSE, "code"=0, "source"=""}} ("Check Connection (Reply Payload)"), "Module ID"=w495, "Is Connected"=w494, "error"=w493) -> (w503:T21)
            n189 = Merge Errors(w499, w493) -> (w501:errorcluster)
            n190 = case "DQMH_FIRE_NOTIFIER" shown="True" w504 {
              tunnel: w505 -> [_ w511]
              tunnel: w503 -> [_ w510]
              frame False {
              }
              frame True {
                n191 = Send Notification(notification=w510, notifier=w511) -> ()  [unwired: 1 in, 2 out]
              }
            }
          }
          frame "Ack Variable Write" {
            n192 = Variant To Data(error in=w528, type=T11 {"Module ID"=-1, "JSON"=""} ("Ack Variable Write Argument"), Variant=w526) -> (data=w524:T11, error out=w527:errorcluster)
            n193 = Unbundle By Name(w524) -> ("JSON"=w513:string)  [unwired: 1 out]
            n194 = Unbundle By Name(w519) -> ("MQTT_Base out"=w518:refnum<class "Client.lvclass">)
            n195 = call "Find Item (as LVtype).vim"("$Path or Item Name"="id", "Data Type and Default Value"="", "JSON"=w513) -> ("Data"=w520:string)  [unwired: 5 in, 3 out]
            n196 = Format Into String(format string="{ \"id\":\"%s\", \"ok\":true, \"result\":{\"written\":true} }", w520) -> (resulting string=w517:string)  [unwired: 2 in, 1 out]
            n197 = call "Find Item (as LVtype).vim"("$Path or Item Name"="reply_to", "Data Type and Default Value"="", "JSON"=w513) -> ("Data"=w512:string)  [unwired: 5 in, 3 out]
            n198 = String To Byte Array(string=w517) -> (unsigned byte array=w516:u8[])
            n199 = call <vilib>:"Publish (Raw Payload).vi"("Binary Payload"=w516, "Topic Name"=w512, "Client in"=w518) -> ()  [unwired: 6 in, 3 out]
          }
          frame "Ack Run Start" {
            n200 = Variant To Data(error in=w546, type=T12 {"Module ID"=-1, "JSON"=""} ("Ack Run Start Argument"), Variant=w544) -> (data=w542:T12, error out=w545:errorcluster)
            n201 = Unbundle By Name(w542) -> ("JSON"=w529:string)  [unwired: 1 out]
            n202 = Unbundle By Name(w532) -> ("MQTT_Base out"=w537:refnum<class "Client.lvclass">)
            n203 = call "Find Item (as LVtype).vim"("$Path or Item Name"="id", "Data Type and Default Value"="", "JSON"=w529) -> ("Data"=w538:string)  [unwired: 5 in, 3 out]
            n204 = Format Into String(format string="{ \"id\":\"%s\", \"ok\":true, \"result\":{\"started\":true} }", w538) -> (resulting string=w531:string)  [unwired: 2 in, 1 out]
            n205 = String To Byte Array(string=w531) -> (unsigned byte array=w536:u8[])
            n206 = call "Find Item (as LVtype).vim"("$Path or Item Name"="reply_to", "Data Type and Default Value"="", "JSON"=w529) -> ("Data"=w533:string)  [unwired: 5 in, 3 out]
            n207 = call <vilib>:"Publish (Raw Payload).vi"("Binary Payload"=w536, "Topic Name"=w533, "Client in"=w537) -> ("error out"=w530:errorcluster)  [unwired: 6 in, 2 out]
            n208 = call "REQ Run Sequence.vi"("error in"=w530, "Run.Start JSON"=w529) -> ()  [unwired: 9 in, 1 out]
          }
          frame "Get Recipe" {
            n209 = property class="Mod Admin"(reference=w552) -> ("Accessors:Module ID"=w553:i32)  [unwired: 1 in, 2 out]
            n210 = Variant To Data(error in=w562, type=T13 {"Module ID"=-1, "Get Recipe JSON"="", "Wait Notifier"=refnum, "wait for reply"=FALSE} ("Get Recipe Argument"), Variant=w560) -> (data=w558:T13, error out=w561:errorcluster)
            n211 = Unbundle By Name(w558) -> ("Get Recipe JSON"=w547:string, "Wait Notifier"=w557:refnum<notifier>, "wait for reply"=w556:bool)  [unwired: 1 out]
            n212 = Unbundle By Name(w550) -> ("MQTT_Base out"=w549:refnum<class "Client.lvclass">)
            n213 = String To Byte Array(string=w547) -> (unsigned byte array=w551:u8[])
            n214 = call <vilib>:"Publish (Raw Payload).vi"("Binary Payload"=w551, "Topic Name"="tmf/st1/query/recipe.fetch", "Client in"=w549) -> ()  [unwired: 6 in, 3 out]
            n215 = disable-structure shown="Disabled" {
              disable-tunnel: [w565 _] -> w555
              disable-tunnel: w553 -> [w563 _]
              frame Disabled {
                n216 = Bundle By Name(cluster=T22 {"Module ID"=-1, "Get Recipe reply JSON"="", "error"={"status"=FALSE, "code"=0, "source"=""}} ("Get Recipe (Reply Payload)"), "Module ID"=w563) -> (w565:T22)  [unwired: 2 in]
              }
              frame Enabled {
              }
            }
            n217 = Merge Errors(w561) -> (w554:errorcluster)
            n218 = case "DQMH_FIRE_NOTIFIER" shown="True" w556 {
              tunnel: w557 -> [_ w567]
              tunnel: w555 -> [_ w566]
              frame False {
              }
              frame True {
                n219 = Send Notification(notification=w566, notifier=w567) -> ()  [unwired: 1 in, 2 out]
              }
            }
          }
          frame "Run Finished" {
            n220 = Variant To Data(error in=w581, type=T14 {"Module ID"=-1, "ts"=0.0, "Run ID"="", "Result"=""} ("Run Finished Argument"), Variant=w579) -> (data=w577:T14, error out=w580:errorcluster)
            n221 = Unbundle By Name(w577) -> ("ts"=w571:dbl, "Run ID"=w570:string, "Result"=w569:string)  [unwired: 1 out]
            n222 = Format Into String(format string="{\n  \"type\": \"run-finished\",\n  \"ts\": %0.1f,\n  \"payload\": {\n    \"run_id\": \"%s\",\n    \"result\": \"%s\"\n  }\n}", w571, w570, w569) -> (resulting string=w568:string)  [unwired: 2 in, 1 out]
            n223 = Unbundle By Name(w573) -> ("MQTT_Base out"=w575:refnum<class "Client.lvclass">)
            n224 = String To Byte Array(string=w568) -> (unsigned byte array=w576:u8[])
            n225 = call <vilib>:"Publish (Raw Payload).vi"("Binary Payload"=w576, "Topic Name"="tmf/st1/event/run-finished", "Client in"=w575) -> ()  [unwired: 6 in, 3 out]
          }
          frame "Test Result" {
            n226 = Variant To Data(error in=w599, type=T15 {"Module ID"=-1, "Test Result payload"={"ts"=0.0, "Run ID"="", "Test name"="", "Expected"="", "Measured"="", "Result"="", "Cycle Time_ms"=0}} ("Test Result Argument"), Variant=w597) -> (data=w595:T15, error out=w598:errorcluster)
            n227 = Unbundle By Name(w595) -> ("Test Result payload.ts"=w588:dbl, "Test Result payload.Run ID"=w587:string, "Test Result payload.Test name"=w586:string, "Test Result payload.Expected"=w585:string, "Test Result payload.Measured"=w584:string, "Test Result payload.Result"=w583:string, "Test Result payload.Cycle Time_ms"=w582:u16)
            n228 = Format Into String(format string="{\n  \"type\": \"test-result\",\n  \"ts\": %0.1f,\n  \"payload\": {\n    \"run_id\": \"%s\",\n    \"test_name\": \"%s\",\n    \"expected\": \"%s\",\n    \"measured\": \"%s\",\n    \"result\": \"%s\",\n    \"cycle_time_ms\": %d\n  }\n}", w588, w587, w586, w585, w584, w583, w582) -> (resulting string=w590:string)  [unwired: 2 in, 1 out]
            n229 = Unbundle By Name(w589) -> ("MQTT_Base out"=w593:refnum<class "Client.lvclass">)
            n230 = String To Byte Array(string=w590) -> (unsigned byte array=w594:u8[])
            n231 = call <vilib>:"Publish (Raw Payload).vi"("Binary Payload"=w594, "Topic Name"="tmf/st1/event/test-result", "Client in"=w593) -> ()  [unwired: 6 in, 3 out]
          }
          frame "---Copy This Frame---" {
            # "Duplicate this frame when creating new messages.  Change this comment in the duplicated frame to describe this message."
            n232 = Merge Errors(w602) -> (w601:errorcluster)
          }
          frame "---Exit and Error Handling---" {
            # "Separator - the following cases handle errors and exit messages."
          }
          frame "Error" {
            # "#DQMH_CodeRecommended - If the module is running in standalone mode (External Launch = FALSE), this code will pop up an error dialog and call the 'Exit' message if an error occurs. Add more fine-grained error management here."
            # "Error - Check the error message data and respond accordingly. This message is sent by the \"Error Handler\" VIs at the end of each loop in this application."
            n233 = property on="Property Node" class="Mod Admin"(reference=w609) -> ("Accessors:External Launch"=w608:bool, "Accessors:Module ID"=w606:i32)  [unwired: 1 in, 2 out]
            n234 = Variant To Data(error in=w616, type=errorcluster {"status"=FALSE, "code"=0, "source"=""} ("error constant"), Variant=w610) -> (data=w605:errorcluster, error out=w614:errorcluster)
            n235 = local write "error out"(w605) -> ()
            n236 = call "Error Reported.vi"("Error"=w605, "Module ID"=w606) -> ()  [unwired: 9 in, 1 out]
            n237 = case shown="False" w608 {
              tunnel: [w621 _] -> w613
              tunnel: w607 -> [w619 _]
              tunnel: w605 -> [w620 _]
              frame False {
                n238 = disable-structure shown="Default" {
                  disable-tunnel: w620 -> [w622 _]
                  frame condition #0 (active) {
                    # "If the module is running standalone, then pop up an error dialog and call the \"Exit\" message."
                    n239 = call <vilib>:"Simple Error Handler.vi"("error in (no error)"=w622) -> ()  [unwired: 4 in, 5 out]
                  }
                  frame condition #1 {
                    # "To prevent the Simple Error Handler VI from being loaded (e.g. when deploying to a Real-Time target), add the Conditional Disable Symbol \"DQMH_Disable_SEH\" to your project and set it to TRUE."
                  }
                }
                n240 = call-poly <vilib>:"Delacor_lib_QMH_Enqueue Message (poly).vi"("Priority Message? (F)"=TRUE, "Message"="Exit", "Message Queue in"=w619) -> ("error out"=w621:errorcluster)  [unwired: 7 in, 1 out]
              }
              frame True {
                # "If the module was launched externally, calling the Error Reported broadcast VI is the only action performed by the \"Error\" message. The module's caller can then process the error appropriately."
              }
            }
            n241 = Merge Errors(w614, w613) -> (w612:errorcluster)
          }
          frame "Simulate MHL Error" {
            # "#DQMH_HowTo The 'Simulate MHL Error' button  illustrates how the MHL handles errors. This event is instructional in nature and can be removed."
            # "Simulate an error occurring at the MHL"
            n242 = property on="Property Node" class="Mod Admin"(reference=w628) -> ("Accessors:Module ID"=w629:i32)  [unwired: 1 in, 2 out]
            n243 = call "Module Name--constant.vi"("Module ID"=w629) -> ("Module Name"=w624:string)  [unwired: 10 in]
            n244 = Format Into String(format string="Simulated error originating at Message Handling Loop in %s", w624) -> (resulting string=w625:string)  [unwired: 2 in, 1 out]
            n245 = call <vilib>:"Error Cluster From Error Code.vi"("show call chain? (False)"=TRUE, "error message (\"\")"=w625, "error code (0)"=5001) -> ("error out"=w631:errorcluster)  [unwired: 6 in]
            n246 = Merge Errors(w633, w631) -> (w632:errorcluster)
          }
          frame "Exit" {
            w641 = 91  # 91: not all Exit messages will have an argument
            w642 = TRUE  # Stop the VI
            # "Release the message queue reference"
            # "#DQMH_CodeNeeded - Add any required cleanup code here."
            # "Exit - Exit the application."
            n247 = Variant To Data(error in=w650, type=T5 {"Module ID"=-1, "Origin"="", "Exit via Stop Module Req?"=FALSE, "Wait for Module to stop?"=FALSE} ("Stop Argument"), Variant=w640) -> (data=w637:T5, error out=w646:errorcluster)
            n248 = call <vilib>:"Clear Errors.vi"("error in (no error)"=w646, "specific error code to clear (0: all)"=w641) -> ("error out"=w649:errorcluster)  [unwired: 4 in, 1 out]
            n249 = property on="Property Node" class="Mod Admin"(reference=w635) -> ("Accessors:Module ID"=w634:i32)  [unwired: 1 in, 2 out]
            n250 = control-ref of="This VI"() -> (w636:refnum<vi>)
            n251 = call-dynamic "Delacor_lib_QMH_Release Message Queue.vi"("error in"=w649, "Message Queue"=w644) -> ("error out"=w648:errorcluster)  [unwired: 9 in]
            n252 = call "Handle Exit.vi"("Stop Argument"=w637, "Module Admin in"=w635, "VI reference"=w636) -> ("error out"=w647:errorcluster, "Wait for Stop?"=w638:bool)  [unwired: 7 in]
            n253 = Merge Errors(w648, w647) -> (w645:errorcluster)
            n254 = call "Error Reported.vi"("Error"=w645, "Module ID"=w634) -> ()  [unwired: 9 in, 1 out]
          }
          frame Default {
            # "'Default' case only runs if there is a message that isn't defined in any of the other cases.  Output a programming error."
            n255 = property on="Property Node" class="Mod Admin"(reference=w658) -> ("Accessors:Module ID"=w657:i32)  [unwired: 1 in, 2 out]
            n256 = call "Module Name--constant.vi"("Module ID"=w657) -> ("Module Name"=w651:string)  [unwired: 10 in]
            n257 = Format Into String(format string="The invalid message string \"%s\" was received in the Message Handling Loop for module \"%s\".", w652, w651) -> (resulting string=w654:string)  [unwired: 2 in, 1 out]
            n258 = call <vilib>:"Error Cluster From Error Code.vi"("show call chain? (False)"=TRUE, "error message (\"\")"=w654, "error code (0)"=1) -> ("error out"=w660:errorcluster)  [unwired: 6 in]
            n259 = Merge Errors(w661, w660) -> (w662:errorcluster)
          }
        }
        n260 = call-dynamic "Delacor_lib_QMH_Error Handler - Message Handling Loop.vi"("error in"=w379, "Message Queue in"=w370) -> ("dup error in"=w376:errorcluster)  [unwired: 8 in, 1 out]
      }
      n261 = while "DQMH_HELPER_LOOP" {
        shift-right: [w69] -> _
        shift-left: 1000 -> [w68]
        shift-right: [w66] -> w47
        shift-left: w46 -> [w67]
        tunnel: w51 -> [w63]
        tunnel: w50 -> [w61]
        shift-right: [w59] -> _
        shift-left: w39 -> [w60]
        shift-right: [w58] -> _
        shift-left: errorcluster {"status"=FALSE, "code"=0, "source"=""} ("error out") -> [w57]
        stop <- w65 stop-if-true
        w62 = "Subscriber Loop"  # DQMH_HELPER_LOOP_NAME
        # "Subscriber Loop"
        n262 = event "DQMH_HELPER_EVENT_STRUCTURE" shown="[0] Timeout" {
          selector: w67 -> [_ _ _ _]
          dyn-events: [_ _ _ _] -> w66
          timeout: w68 -> [_ _ _ _]
          tunnel: w68 -> [w83 w102 w132 w140]
          tunnel: [w83 w102 w132 w140] -> w69
          tunnel: [_ _ w129 _] -> w65
          tunnel: [_ w94 errorcluster {"status"=FALSE, "code"=0, "source"=""} ("error constant") _] -> w64
          tunnel: w63 -> [_ _ _ _]
          tunnel: w61 -> [w81 w93 w130 w136]
          tunnel: w60 -> [w82 w100 w127 w139]
          tunnel: [w82 w100 w127 w138] -> w59
          tunnel: [w71 w94 w126 w133] -> w58
          tunnel: w57 -> [w77 w95 w126 w133]
          event Timeout {
            n263 = event-data() -> ()  [unwired: 1 in, 1 out]
            n264 = Unbundle By Name(w82) -> ("MQTT_Base out"=w76:refnum<class "Client.lvclass">)
            n265 = property class="Mod Admin"(reference=w81) -> ("Accessors:Module ID"=w79:i32)  [unwired: 1 in, 2 out]
            n266 = Format Into String(format string="tmf/st%d/status" ("Topic Name"), w79) -> (resulting string=w70:string)  [unwired: 2 in, 1 out]
            n267 = call <vilib>:"isConnected.vi"("error in (no error)"=w77, "Client in"=w76) -> ("error out"=w73:errorcluster, "connected"=w72:bool, "Client out"=w74:refnum<class "Client.lvclass">)  [unwired: 7 in]
            n268 = String To Byte Array(string="{\"state\":\"online\"}") -> (unsigned byte array=w75:u8[])
            n269 = case shown="True" w72 {
              tunnel: w79 -> [w85 _]
              tunnel: w75 -> [_ w91]
              tunnel: w74 -> [_ w90]
              tunnel: w73 -> [w84 w89]
              tunnel: [w84 w88] -> w71
              tunnel: w70 -> [_ w87]
              frame False {
                n270 = call "Status Updated.vi"("Status"="Server not connected", "Module ID"=w85) -> ()  [unwired: 9 in, 1 out]
              }
              frame True {
                n271 = call <vilib>:"Publish (Raw Payload).vi"("error in (no error)"=w89, "Binary Payload"=w91, "Topic Name"=w87, "Client in"=w90) -> ("error out"=w88:errorcluster)  [unwired: 5 in, 2 out]
              }
            }
          }
          event User Event {
            n272 = event-data() -> ("PUBLISH"=w101:refnum<class "PUBLISH.lvclass">)  [unwired: 1 in]
            n273 = Unbundle By Name(w100) -> ("MQTT_Base out"=w98:refnum<class "Client.lvclass">)
            n274 = property class="Mod Admin"(reference=w93) -> ("Accessors:Module ID"=w92:i32)  [unwired: 1 in, 2 out]
            n275 = call <vilib>:"isConnected.vi"("error in (no error)"=w95, "Client in"=w98) -> ("error out"=w96:errorcluster, "connected"=w99:bool, "Client out"=w97:refnum<class "Client.lvclass">)  [unwired: 7 in]
            n276 = case shown="True" w99 {
              tunnel: w101 -> [_ w114]
              tunnel: w97 -> [_ w113]
              tunnel: w96 -> [w105 w111]
              tunnel: [w105 w109] -> w94
              tunnel: w92 -> [w104 w108]
              frame False {
                n277 = call "Status Updated.vi"("Status"="Disconnected", "Module ID"=w104) -> ()  [unwired: 9 in, 1 out]
              }
              frame True {
                n278 = call <vilib>:"getTopicName.vi"("PUBLISH in"=w114) -> ("PUBLISH out"=w115:refnum<class "PUBLISH.lvclass">)  [unwired: 8 in, 2 out]
                n279 = call <vilib>:"Decode Application Message (Raw).vi"("error in (no error)"=w111, "PUBLISH"=w115, "Client in"=w113) -> ("error out"=w110:errorcluster, "Payload"=w112:u8[], "Topic"=w106:string)  [unwired: 5 in, 1 out]
                "Topic" <- w106
                n280 = Byte Array To String(unsigned byte array=w112) -> (string=w107:string)
                "payload" <- w107
                n281 = case shown="\"tmf/st1/cmd/variable.write\"" w106 {
                  tunnel: w110 -> [w116 w120 w124 w125]
                  tunnel: [w116 w119 w123 w125] -> w109
                  tunnel: w108 -> [_ w118 w122 _]
                  tunnel: w107 -> [_ w117 w121 _]
                  frame Default {
                  }
                  frame "tmf/st1/cmd/variable.write" {
                    n282 = call "Ack Variable Write.vi"("error in"=w120, "JSON"=w117, "Module ID"=w118) -> ("error out"=w119:errorcluster)  [unwired: 8 in]
                  }
                  frame "tmf/st1/cmd/run.start" {
                    n283 = call "Ack Run Start.vi"("error in"=w124, "JSON"=w121, "Module ID"=w122) -> ("error out"=w123:errorcluster)  [unwired: 8 in]
                  }
                  frame "tmf/st1/query/resp/lv-1" {
                  }
                }
              }
            }
          }
          event User Event {
            n284 = event-data() -> ("Module ID"=w128:i32)  [unwired: 1 in]
            n285 = call "Addressed to This Module.vi"("Module ID from Argument"=w128, "Module Admin"=w130) -> ("Addressed to this instance?"=w129:bool)  [unwired: 8 in, 1 out]
          }
          event User Event {
            n286 = event-data() -> ("Module ID"=w135:i32, "Client out"=w137:refnum<class "Client.lvclass">)  [unwired: 1 in]
            n287 = call "Addressed to This Module.vi"("Module ID from Argument"=w135, "Module Admin"=w136) -> ("Addressed to this instance?"=w134:bool)  [unwired: 8 in, 1 out]
            n288 = case shown="False" w134 {
              tunnel: w139 -> [w141 w144]
              tunnel: [w141 w143] -> w138
              tunnel: w137 -> [_ w142]
              frame False {
              }
              frame True {
                n289 = Bundle By Name(cluster=w144, "MQTT_Base out"=w142) -> (w143:T23)
              }
            }
          }
        }
        n290 = call-dynamic "Delacor_lib_QMH_Error Handler - Helper Loop.vi"("Error Debug"=w62, "error in"=w64, "Message Queue in"=w63) -> ()  [unwired: 7 in, 2 out]
      }
      n291 = Unregister For Events(event registration refnum=w47) -> ()  [unwired: 1 in, 1 out]
    }
    frame Error {
      n292 = call "Synchronize Caller Events.vi"("Module Admin"=w666) -> ("Module Admin out"=w665:refnum<class "Delacor_lib_QMH_Cloneable Module Admin.lvclass">)  [unwired: 9 in, 1 out]
      n293 = property on="Property Node" class="Mod Admin"(reference=w665) -> ("Accessors:Module ID"=w664:i32)  [unwired: 1 in, 2 out]
      n294 = call-dynamic "Delacor_lib_QMH_Release Message Queue.vi"("error in"=w672, "Message Queue"=w663) -> ("error out"=w671:errorcluster)  [unwired: 9 in]
      n295 = call "Module Name--constant.vi"("Module ID"=w664) -> ("Module Name"=w669:string)  [unwired: 10 in]
      n296 = Format Into String(format string="An error occurred during initialization. %s is no longer running.", w669) -> (resulting string=w667:string)  [unwired: 2 in, 1 out]
      n297 = call "Error Reported.vi"("Additional Information"=w667, "Error"=w671, "Module ID"=w664) -> ()  [unwired: 8 in, 1 out]
    }
  }
  n298 = Merge Errors(w35, w34) -> (w36:errorcluster)
  n299 = call "Close Module.vi"("error in"=w36, "Wait for stop?"=w22, "Module Admin in"=w24) -> ("error out"=w32:errorcluster, "External Launch"=w21:bool, "Module Admin out"=w23:refnum<class "Delacor_lib_QMH_Cloneable Module Admin.lvclass">)  [unwired: 6 in]
  n300 = Unregister For Events(event registration refnum=w28, error in=w32) -> (error out=w2:errorcluster)
  "error out" <- w2
  n301 = local write "Module Admin"(w23) -> ()
  n302 = case "External Launch?" shown="True" w21 {
    tunnel: w2 -> [_ w673]
    frame False {
    }
    frame True {
      n303 = case shown="No Error" w673 {
        frame No Error {
          n304 = disable-structure shown="Disabled" {
            frame Disabled {
              n305 = invoke class="VI" method="FP.Close"() -> ()  [unwired: 3 in, 3 out]
            }
            frame Enabled {
            }
          }
        }
        frame Error {
          n306 = disable-structure shown="Default" {
            frame condition #0 (active) {
              n307 = invoke class="VI" method="FP.Open"("Activate"=TRUE ("Activate?")) -> ()  [unwired: 4 in, 5 out]
            }
            frame condition #1 {
              # "Don't show panel on error if running inside a built EXE."
            }
          }
        }
      }
    }
  }
  n308 = flat-sequence {
    tunnel: w2 -> [w676]
    tunnel: w5 -> [w675]
    frame #0 {
      n309 = call <vilib>:"Stop.vi"("error in (no error)"=w676, "MQTT_Base in"=w675) -> ("error out"=w678:errorcluster, "MQTT_Base out"=w677:refnum<class "Client.lvclass">)  [unwired: 7 in, 1 out]
      n310 = call <vilib>:"Destroy.vi"("error in (no error)"=w678, "MQTT_Base in"=w677) -> ()  [unwired: 8 in, 2 out]
    }
  }
  n311 = case shown="False" w1 {
    tunnel: w2 -> [_ _]
    frame False {
      n312 = call "Stop Module.vi"() -> ()  [unwired: 11 in, 1 out]
    }
    frame True {
    }
  }
